vi "Replace_row (SubVI).vi"(9 "replace_row":u32, 10 "substring (\"\")":string, 11 "StringIn":string) -> (3 "StringOut":string)   [LabVIEW 2017]
panel:
  out "offset past replacement":i32
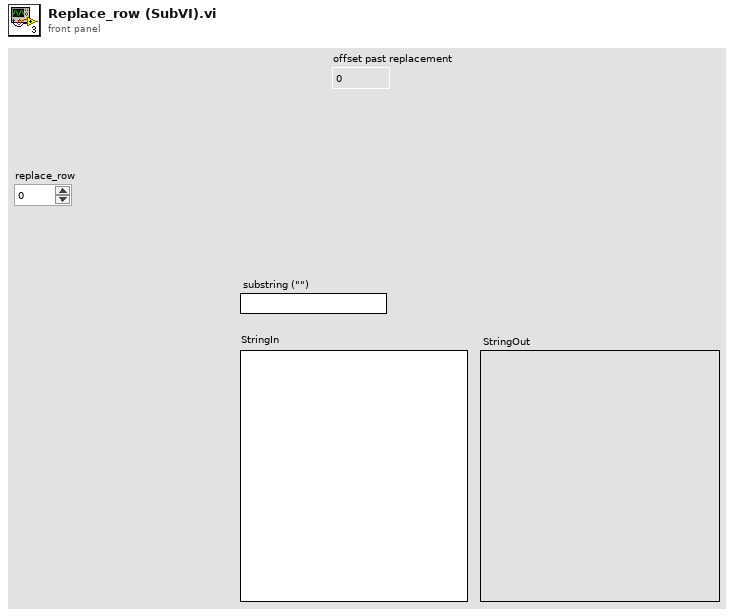
[diagram p1: front panel]
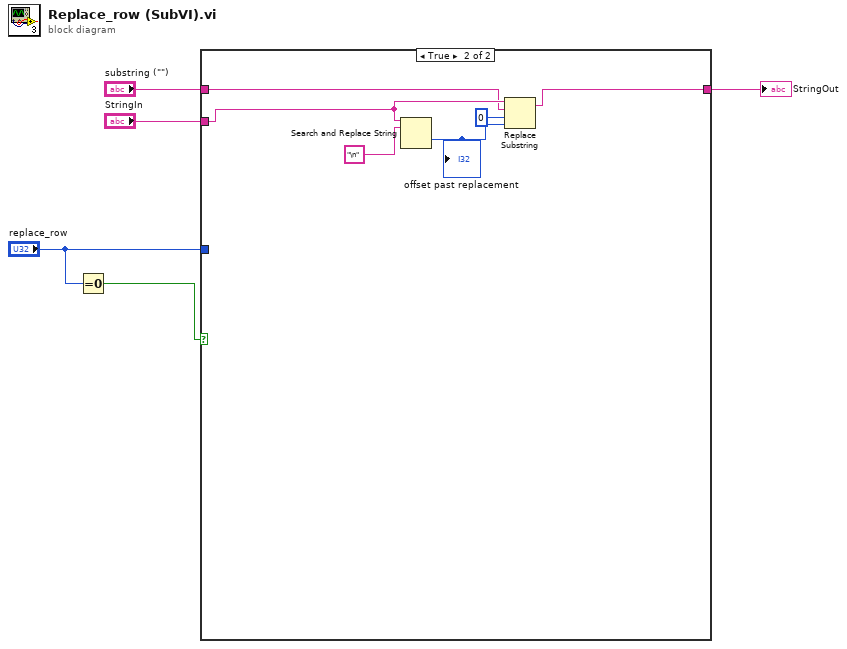
[diagram p0: block diagram]
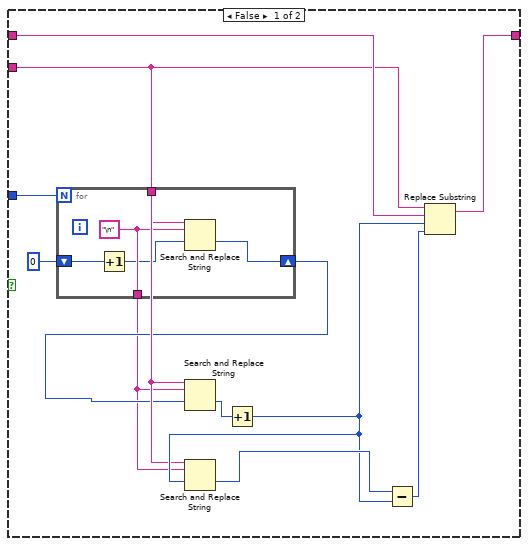
[diagram p2: hidden frame]
diagram:
  n1 = Equal To 0?(x="replace_row") -> (x = 0?=w1:bool)
  n2 = case shown="True" w1 {
    tunnel: [w15 w25] -> w5
    tunnel: "substring (\"\")" -> [w11 w22]
    tunnel: "StringIn" -> [w10 w23]
    tunnel: "replace_row" -> [w6 _]
    frame False {
      n3 = for {
        N: w6 -> [_]
        tunnel: w10 -> [w21]
        tunnel: [w20] -> w8
        shift-right: [w19] -> w9
        shift-left: 0 -> [w18]
        w20 = "\n" ("search string")
        n4 = Increment(x=w18) -> (x+1=w17:i32)
        n5 = Search and Replace String(input string=w21, search string=w20, offset=w17) -> (offset past replacement=w19:i32)  [unwired: 5 in, 3 out]
      }
      n6 = Search and Replace String(input string=w10, search string=w8, offset=w9) -> (offset past replacement=w16:i32)  [unwired: 5 in, 3 out]
      n7 = Increment(x=w16) -> (x+1=w12:i32)
      n8 = Search and Replace String(input string=w10, search string=w8, offset=w12) -> (offset past replacement=w13:i32)  [unwired: 5 in, 3 out]
      n9 = Subtract(x=w13, y=w12) -> (x-y=w14:i32)
      n10 = Replace Substring(2:w14, 3:w12, 4:w11, 5:w10) -> (1:w15:string)  [unwired: 1 out]
    }
    frame True {
      n11 = Search and Replace String(input string=w23, search string="\n") -> (offset past replacement=w26:i32)  [unwired: 6 in, 3 out]
      "offset past replacement" <- w26
      n12 = Replace Substring(2:w26, 3:0 ("offset (0)"), 4:w22, 5:w23) -> (1:w25:string)  [unwired: 1 out]
    }
  }
  "StringOut" <- w5
